vi "SIMPS 2.5.vi"() -> ()   [LabVIEW 2020]
uses:
  <vilib>/Utility/NIReport.llb/Report Type.ctl
  <vilib>/Analysis/1siggen.llb/Ramp Pattern by Samples.vi
  <vilib>/measure/maspectr.llb/FFT Spectrum (Mag-Phase) for 1 Chan.vi
  <vilib>/addons/_office/excel.llb/Excel Easy Table (num).vi
  <vilib>/Utility/NIReport.llb/NI_report.lvclass
  <vilib>/measure/NI_MABase.lvlib
  <vilib>/Analysis/NI_AALBase.lvlib
  <vilib>/Utility/NIReport.llb/NI_ReportGenerationCore.lvlib
  <vilib>/Utility/NIReport.llb/Excel/NI_Excel.lvclass
  <vilib>/addons/_office/NI_ReportGenerationToolkit.lvlib
  <vilib>/measure/NI_MAPro.lvlib
panel:
  out "Analysis Data":dynamicdata[](array[waveform])
  in  "Trigger Measurement":bool
  out "Device Mode":string
  in  "Trigger Program":bool
  in  "Generate Results Report":bool
  out "Function Generator Waveform":waveform(dbl)
  out "DUT Waveform":waveform(dbl)
  out "Gain (Multiplier)":dbl
  out "Slew Rate (V/s)":dbl
  out "Overshoot (%)":dbl
  out "Preshoot (%)":dbl
  out "Frequency (Hz) 2":dbl
  out "SINAD (dB)":dbl
  out "Amplitude (Vpk-pk)":dbl
  out "MEAN (DC V)":dbl
  out "THD (%)":dbl
  out "Negative Peak (Vpk)":dbl
  out "Positive Peak (Vpk)":dbl
  out "RMS (Vrms)":dbl
  in  "PS Update":bool
  out "Actual Voltage":dbl
  in  "PS State":bool
  out "PS Enabled":bool
  in  "Power Supply (V)":dbl=1.6 min=1.6 max=59.3
  in  "Range Selection":u8=1 min=1 max=4 step=1
  out "Current Range":u8
  in  "FG State":bool
  out "FG Enabled":bool
  in  "Duty Cycle (%)":dbl=50.0
  in  "Phase (Degrees)":dbl
  in  "DC Offset (V)":dbl min=-5.0 max=5.0 step=0.1
  in  "Frequency (Hz)":dbl=1000.0 min=1.0 max=2000000.0 step=1.0
  in  "Amplitude (V)":dbl=5.0 min=0.0 max=10.0 step=0.1
  in  "Function Selection":enum16{"Sine", "Square", "Triangle", "Ramp"}(ring)
  out "Measurement Waveforms":waveform(dbl)[](graph)
  out "FFT Magnitude":cluster{"f0":dbl, "df":dbl, "magnitude":dbl[]}(graph)
  out "FFT Phase":cluster{"f0":dbl, "df":dbl, "phase":dbl[]}(graph)
  out "Function Generator Waveform Graph":waveform(dbl)(graph)
  # "SIMPS ATE - LabVIEW Interface"
  # "Note: The device needs to be in the programming mode to program."
  # "Test Results & Analysis"
  # "Gain"
  # "Distortion Measurements"
  # "Level Measurements"
  # "Timing/Transition Measurements"
  # "DC Power Supply"
  # "The voltage entry is rounded to the nearest 10-bit value."
  # "Measurement"
  # "Select a proper range for the measurement of the DUT."
  # "1: 0-4V, 2: 4-10V, 3: 10-20V, 4: 20-60V"
  # "Function Generator"
  # "Note: The device must be programmed to change the function generator output."
  # "Eric Birtcil, Travis Draney, Nick Peck, Kyle Roy"
  # "Team Unlimited Power's Capstone Project"
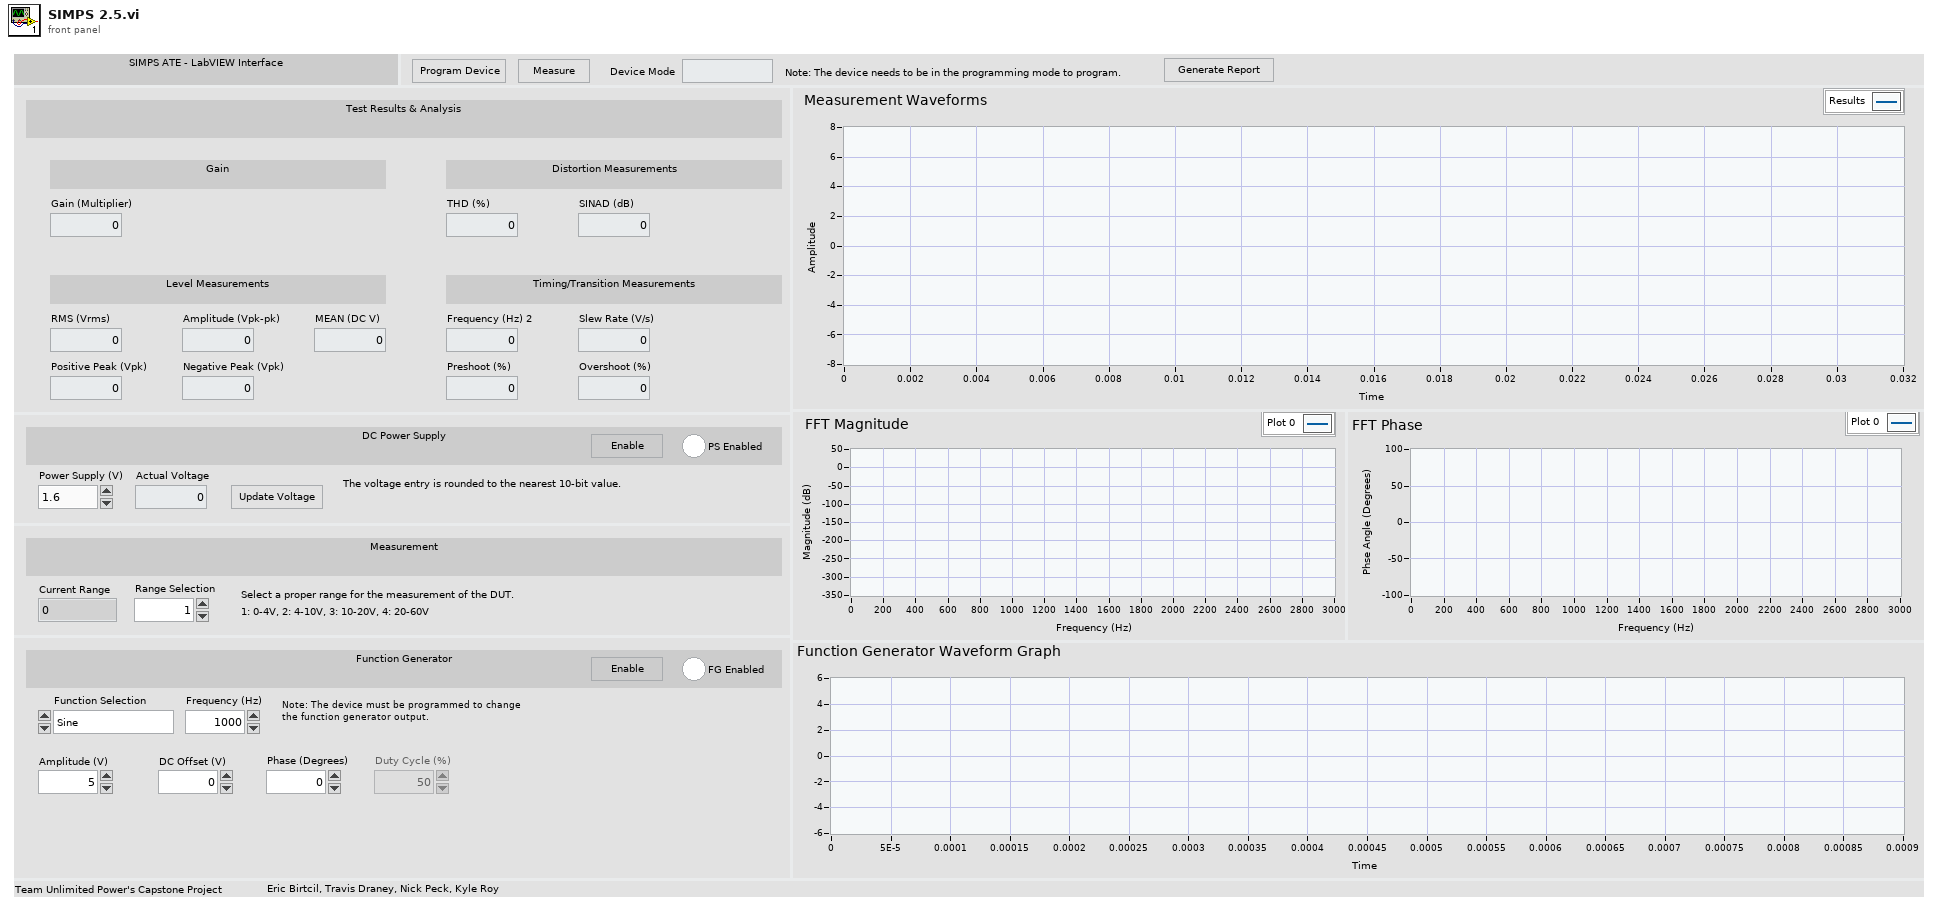
[diagram p1: front panel]
types:
  T1 = typedef "NI_ReportGenerationCore.lvlib/Report Type.ctl" = enum16{"HTML", "Word", "Excel"}
  T2 = enum8{"Enabled", "Disabled", "Disabled and Grayed Out"}
  T3 = cluster{"dB On (F)":bool, "unwrap phase (F)":bool, "convert to degree (F)":bool}
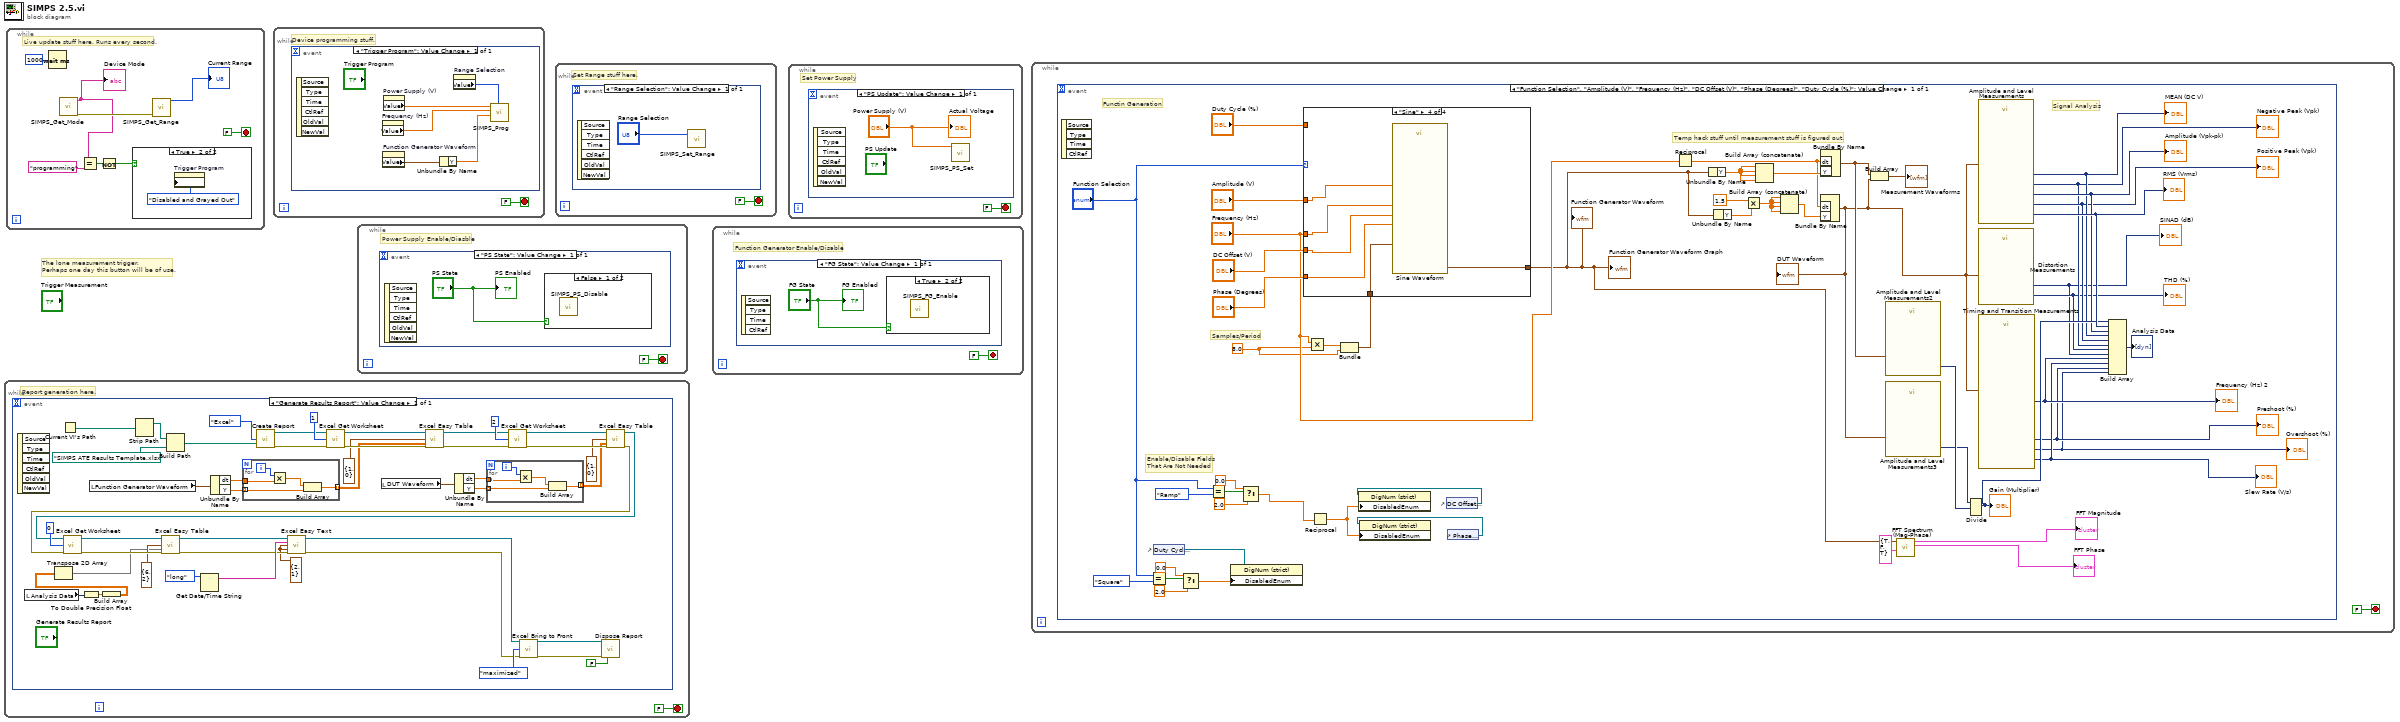
[diagram p0: block diagram]
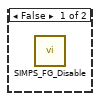
[diagram p2: hidden frame]
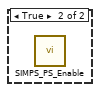
[diagram p3: hidden frame]
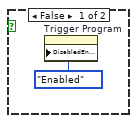
[diagram p4: hidden frame]
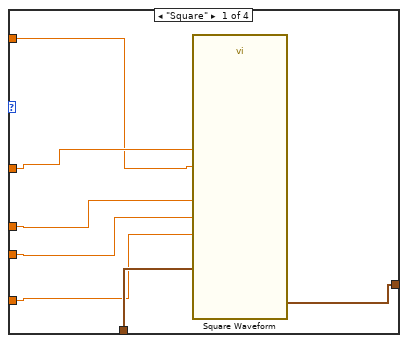
[diagram p5: hidden frame]
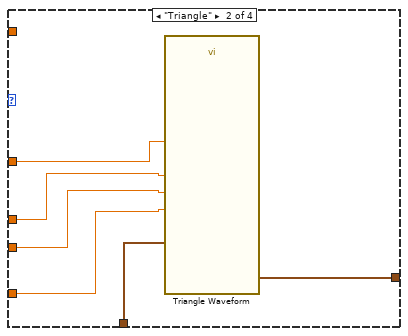
[diagram p6: hidden frame]
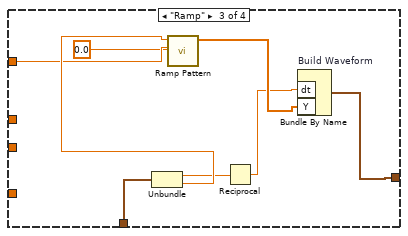
[diagram p7: hidden frame]
diagram:
  # "The lone measurement trigger.\nPerhaps one day this button will be of use."
  n1 = while {
    stop <- FALSE stop-if-true
    # "Report generation here."
    n2 = event shown="[0] \"Generate Results Report\": Value Change" {
      selector: _ -> [_]
      dyn-events: _ -> [_]
      timeout: _ -> [_]
      event "Generate Results Report": Value Change {
        w4 = cluster{"row":i32, "column":i32} {"row"=2, "column"=1} ("start (-1, -1)")
        n3 = event-data() -> ()  [unwired: 1 in, 6 out]
        n4 = local read "Analysis Data"() -> (w13:dynamicdata[])
        n5 = Current VI's Path() -> (path=w33:path)
        n6 = To Double Precision Float(number=w13) -> (double precision float=w14:dbl[])
        n7 = local read "Function Generator Waveform"() -> (w36:waveform(dbl))
        n8 = Build Array(w14) -> (w2:dbl[][])
        n9 = Transpose 2D Array(2D array=w2) -> (transposed array=w3:dbl[][])
        n10 = Strip Path(path=w33) -> (stripped path=w34:path)  [unwired: 1 out]
        n11 = Build Path(base path=w34, name or relative path=path "SIMPS ATE Results Template.xlsx") -> (appended path=w45:path)
        n12 = Get Date/Time String(date format (0)=enum16{"short", "long", "abbreviated"}."long") -> (date string=w9:string)  [unwired: 2 in, 1 out]
        n13 = Unbundle By Name(w36) -> ("dt"=w38:dbl, "Y"=w37:dbl[])
        n14 = for {
          tunnel: w38 -> [w57]
          tunnel: w37 -> [w55] mode=indexing
          tunnel: [w53] -> w30 mode=indexing
          i -> [w56]
          n15 = Multiply(x=w56, y=w57) -> (x*y=w54:dbl)
          n16 = Build Array(w54, w55) -> (w53:dbl[])
        }
        n17 = call <vilib>:"Create Report.vi"("report type"=Report_Type."Excel", "template (empty)"=w45) -> ("report out"=w43:refnum<class "NI_report.lvclass">, "error out"=w42:errorcluster)  [unwired: 12 in]
        n18 = call <vilib>:"Excel Get Worksheet.vi"("report in"=w43, "worksheet index (0)"=1, "error in (no error)"=w42) -> ("report out"=w31:refnum<class "NI_report.lvclass">, "error out"=w32:errorcluster)  [unwired: 11 in]
        n19 = local read "DUT Waveform"() -> (w19:waveform(dbl))
        n20 = call-poly <vilib>:"Excel Easy Table.vi"("report in"=w31, "start (0, 0)"=cluster{"row":i32, "column":i32} {"row"=1, "column"=0}, "text data"=w30, "error in (no error)"=w32) -> ("report out"=w21:refnum<class "NI_report.lvclass">, "error out"=w20:errorcluster)  [unwired: 7 in, 3 out]
        n21 = Unbundle By Name(w19) -> ("dt"=w28:dbl, "Y"=w27:dbl[])
        n22 = for {
          tunnel: w28 -> [w52]
          tunnel: w27 -> [w50] mode=indexing
          tunnel: [w48] -> w24 mode=indexing
          i -> [w51]
          n23 = Multiply(x=w51, y=w52) -> (x*y=w49:dbl)
          n24 = Build Array(w49, w50) -> (w48:dbl[])
        }
        n25 = call <vilib>:"Excel Get Worksheet.vi"("report in"=w21, "worksheet index (0)"=2, "error in (no error)"=w20) -> ("report out"=w25:refnum<class "NI_report.lvclass">, "error out"=w26:errorcluster)  [unwired: 11 in]
        n26 = call-poly <vilib>:"Excel Easy Table.vi"("report in"=w25, "start (0, 0)"=cluster{"row":i32, "column":i32} {"row"=1, "column"=0}, "text data"=w24, "error in (no error)"=w26) -> ("report out"=w11:refnum<class "NI_report.lvclass">, "error out"=w12:errorcluster)  [unwired: 7 in, 3 out]
        n27 = call <vilib>:"Excel Get Worksheet.vi"("report in"=w11, "worksheet index (0)"=0, "error in (no error)"=w12) -> ("report out"=w17:refnum<class "NI_report.lvclass">, "error out"=w18:errorcluster)  [unwired: 11 in]
        n28 = call-poly <vilib>:"Excel Easy Table.vi"("report in"=w17, "start (0, 0)"=cluster{"row":i32, "column":i32} {"row"=6, "column"=2}, "text data"=w3, "error in (no error)"=w18) -> ("report out"=w8:refnum<class "NI_report.lvclass">, "error out"=w7:errorcluster)  [unwired: 7 in, 3 out]
        n29 = call <vilib>:"Excel Easy Text.vi"("report in"=w8, "text"=w9, "start (-1, -1)"=w4, "end (-1, -1)"=w4, "error in (no error)"=w7) -> ("report out"=w6:refnum<class "NI_report.lvclass">, "error out"=w5:errorcluster)  [unwired: 6 in, 3 out]
        n30 = call <vilib>:"Excel Bring to Front.vi"("report in"=w6, "window state (maximized)"=enum16{"maximized", "minimized", "normal"}."maximized", "error in (no error)"=w5) -> ("report out"=w40:refnum<class "NI_report.lvclass">, "error out"=w39:errorcluster)  [unwired: 11 in]
        n31 = call-dynamic "Dispose Report.vi"("report in"=w40, "error in (no error)"=w39, "close report? (T)"=FALSE) -> ()  [unwired: 12 in, 1 out]
      }
    }
  }
  n32 = while {
    stop <- FALSE stop-if-true
    # "Live update stuff here. Runs every second."
    n33 = Wait (ms)(milliseconds to wait=u32 1000) -> ()  [unwired: 1 out]
    n34 = call "SIMPS_Get_Mode.vi"() -> ("error out"=w62:errorcluster, "String"=w61:string)  [unwired: 10 in]
    "Device Mode" <- w61
    n35 = Equal?(x=w61, y="programming") -> (x = y?=w59:bool)
    n36 = Not(x=w59) -> (.not. x?=w58:bool)
    n37 = case shown="True" w58 {
      frame False {
        n38 = property on="Trigger Program" class="Bool"("DisabledEnum"=T2."Enabled" ("Disabled")) -> ()  [unwired: 2 in, 2 out]
      }
      frame True {
        n39 = property on="Trigger Program" class="Bool"("DisabledEnum"=T2."Disabled and Grayed Out" ("Disabled")) -> ()  [unwired: 2 in, 2 out]
      }
    }
    n40 = call "SIMPS_Get_Range.vi"("error in (no error)"=w62) -> ("Numeric"=→"Current Range":u8)  [unwired: 9 in, 1 out]
  }
  n41 = while {
    stop <- FALSE stop-if-true
    # "Device programming stuff."
    n42 = event shown="[0] \"Trigger Program\": Value Change" {
      selector: _ -> [_]
      dyn-events: _ -> [_]
      timeout: _ -> [_]
      event "Trigger Program": Value Change {
        n43 = event-data() -> ()  [unwired: 1 in, 6 out]
        n44 = property on="Frequency (Hz)" class="DigNum (strict)"() -> ("Value"=w71:dbl)  [unwired: 2 in, 2 out]
        n45 = property on="Function Generator Waveform" class="WFD (strict)"() -> ("Value"=w73:waveform(dbl))  [unwired: 2 in, 2 out]
        n46 = property on="Power Supply (V)" class="DigNum (strict)"() -> ("Value"=w72:dbl)  [unwired: 2 in, 2 out]
        n47 = Unbundle By Name(w73) -> ("Y"=w69:dbl[])
        n48 = property on="Range Selection" class="DigNum (strict)"() -> ("Value"=w70:u8)  [unwired: 2 in, 2 out]
        n49 = call "SIMPS_Prog.vi"("Range"=w70, "Waveform Values"=w69, "Frequency"=w71, "PS_Voltage"=w72) -> ()  [unwired: 7 in, 1 out]
      }
    }
  }
  n50 = while {
    stop <- FALSE stop-if-true
    # "Power Supply Enable/Diasble"
    n51 = event shown="[0] \"PS State\": Value Change" {
      selector: _ -> [_]
      dyn-events: _ -> [_]
      timeout: _ -> [_]
      event "PS State": Value Change {
        n52 = event-data() -> ()  [unwired: 1 in, 6 out]
        n53 = case shown="False" "PS State" {
          frame False {
            n54 = call "SIMPS_PS_Disable.vi"() -> ()  [unwired: 11 in, 1 out]
          }
          frame True {
            n55 = call "SIMPS_PS_Enable.vi"() -> ()  [unwired: 11 in, 1 out]
          }
        }
        "PS Enabled" <- "PS State"
      }
    }
  }
  n56 = while {
    stop <- FALSE stop-if-true
    # "Set Range stuff here."
    n57 = event shown="[0] \"Range Selection\": Value Change" {
      selector: _ -> [_]
      dyn-events: _ -> [_]
      timeout: _ -> [_]
      event "Range Selection": Value Change {
        n58 = event-data() -> ()  [unwired: 1 in, 6 out]
        n59 = call "SIMPS_Set_Range.vi"("Range"="Range Selection") -> ()  [unwired: 10 in, 1 out]
      }
    }
  }
  n60 = while {
    stop <- FALSE stop-if-true
    # "Function Generator Enable/Disable"
    n61 = event shown="[0] \"FG State\": Value Change" {
      selector: _ -> [_]
      dyn-events: _ -> [_]
      timeout: _ -> [_]
      event "FG State": Value Change {
        n62 = event-data() -> ()  [unwired: 1 in, 4 out]
        n63 = case shown="True" "FG State" {
          frame False {
            n64 = call "SIMPS_FG_Disable.vi"() -> ()  [unwired: 11 in, 1 out]
          }
          frame True {
            n65 = call "SIMPS_FG_Enable.vi"() -> ()  [unwired: 11 in, 1 out]
          }
        }
        "FG Enabled" <- "FG State"
      }
    }
  }
  n66 = while {
    stop <- FALSE stop-if-true
    # "Set Power Supply"
    n67 = event shown="[0] \"PS Update\": Value Change" {
      selector: _ -> [_]
      dyn-events: _ -> [_]
      timeout: _ -> [_]
      event "PS Update": Value Change {
        n68 = event-data() -> ()  [unwired: 1 in, 6 out]
        n69 = call "SIMPS_PS_Set.vi"("PS_Voltage"="Power Supply (V)") -> ()  [unwired: 10 in, 1 out]
        "Actual Voltage" <- "Power Supply (V)"
      }
    }
  }
  n70 = while {
    stop <- FALSE stop-if-true
    n71 = event shown="[0] \"Function Selection\", \"Amplitude (V)\", \"Frequency (Hz)\", \"DC Offset (V)\", \"Phase (Degrees)\", \"Duty Cycle (%)\": Value Change" {
      selector: _ -> [_]
      dyn-events: _ -> [_]
      timeout: _ -> [_]
      event "Function Selection", "Amplitude (V)", "Frequency (Hz)", "DC Offset (V)", "Phase (Degrees)", "Duty Cycle (%)": Value Change {
        w83 = 8.0 ("Samples/Period")
        # "Temp hack stuff until measurement stuff is figured out."
        # "Samples/Period"
        # "Enable/Disable Fields\nThat Are Not Needed"
        # "Signal Analysis"
        # "Functin Generation"
        n72 = event-data() -> ()  [unwired: 1 in, 4 out]
        n73 = Equal?(x="Function Selection", y=enum16{"Sine", "Square", "Triangle", "Ramp"}."Square") -> (x = y?=w128:bool)
        n74 = control-ref of="Duty Cycle (%)"() -> (w124:refnum<vi>)
        n75 = Select(t=0.0, s=w128, f=2.0) -> (s? t:f=w123:dbl)
        n76 = Equal?(x="Function Selection", y=enum16{"Sine", "Square", "Triangle", "Ramp"}."Ramp") -> (x = y?=w121:bool)
        n77 = property class="DigNum (strict)"(reference=w124, "DisabledEnum"=w123) -> ()  [unwired: 1 in, 2 out]
        n78 = Select(t=0.0, s=w121, f=2.0) -> (s? t:f=w117:dbl)
        n79 = Multiply(x="Frequency (Hz)", y=w83) -> (x*y=w133:dbl)
        n80 = Reciprocal(x=w117) -> (1/x=w116:dbl)
        n81 = Bundle(w133, "Samples/Period"=w83) -> (w134:cluster{dbl, "Samples/Period":dbl})  [unwired: 1 in]
        n82 = case shown="\"Sine\"" "Function Selection" {
          tunnel: [w141 w147 w155 w156] -> w85
          tunnel: "Amplitude (V)" -> [w136 w146 w149 w157]
          tunnel: "Frequency (Hz)" -> [w137 w145 _ w158]
          tunnel: "DC Offset (V)" -> [w138 w144 _ w159]
          tunnel: "Phase (Degrees)" -> [w139 w143 _ w160]
          tunnel: w134 -> [w140 w142 w154 w161]
          tunnel: "Duty Cycle (%)" -> [w135 _ _ _]
          frame "Square" {
            n83 = call <vilib>:"Square Waveform.vi"("duty cycle (%)"=w135, "offset"=w138, "sampling info"=w140, "phase"=w139, "amplitude"=w136, "frequency"=w137) -> ("signal out"=w141:waveform(dbl))  [unwired: 4 in, 1 out]
          }
          frame "Triangle" {
            n84 = call <vilib>:"Triangle Waveform.vi"("offset"=w144, "sampling info"=w142, "phase"=w143, "amplitude"=w146, "frequency"=w145) -> ("signal out"=w147:waveform(dbl))  [unwired: 5 in, 1 out]
          }
          frame "Ramp" {
            n85 = Unbundle(w154) -> (w151:dbl, "Samples/Period"=w153:dbl)
            n86 = call-poly <vilib>:"Ramp Pattern.vi"("start"=0.0, "end"=w149, "samples"=w153) -> ("Ramp Pattern"=w152:dbl[])  [unwired: 7 in, 1 out]
            n87 = Reciprocal(x=w151) -> (1/x=w150:dbl)
            n88 = Bundle By Name "Build Waveform"("dt"=w150, "Y"=w152) -> (w155:waveform(dbl))  [unwired: 1 in]
          }
          frame "Sine" {
            n89 = call <vilib>:"Sine Waveform.vi"("offset"=w159, "sampling info"=w161, "phase"=w160, "amplitude"=w157, "frequency"=w158) -> ("signal out"=w156:waveform(dbl))  [unwired: 5 in, 1 out]
          }
        }
        "Function Generator Waveform Graph" <- w85
        "Function Generator Waveform" <- w85
        n90 = control-ref of="DC Offset (V)"() -> (w115:refnum<vi>)
        n91 = property class="DigNum (strict)"(reference=w115, "DisabledEnum"=w116) -> ()  [unwired: 1 in, 2 out]
        n92 = control-ref of="Phase (Degrees)"() -> (w114:refnum<vi>)
        n93 = property class="DigNum (strict)"(reference=w114, "DisabledEnum"=w116) -> ()  [unwired: 1 in, 2 out]
        n94 = Reciprocal(x="Frequency (Hz)") -> (1/x=w106:dbl)
        n95 = Unbundle By Name(w85) -> ("Y"=w111:dbl[])
        n96 = Unbundle By Name(w85) -> ("Y"=w110:dbl[])
        n97 = Multiply(x=1.5, y=w110) -> (x*y=w108:dbl[])
        n98 = Build Array (concatenate)(w111, w111, w111, w111) -> (w112:dbl[])
        n99 = Build Array (concatenate)(w108, w108, w108, w108) -> (w105:dbl[])
        n100 = Bundle By Name("dt"=w106, "Y"=w105) -> (w88:waveform(dbl))  [unwired: 1 in]
        "DUT Waveform" <- w88
        n101 = Bundle By Name("dt"=w106, "Y"=w112) -> (w104:waveform(dbl))  [unwired: 1 in]
        n102 = Build Array(w104, w88) -> (→"Measurement Waveforms":waveform(dbl)[])
        n103 = call "Amplitude and Level Measurements2"("Signals"=w104) -> ("Peak to Peak"=w103:dynamicdata)  [unwired: 13 in, 1 out]
        n104 = call "Amplitude and Level Measurements3"("Signals"=w88) -> ("Peak to Peak"=w102:dynamicdata)  [unwired: 13 in, 1 out]
        n105 = call-poly <vilib>:"FFT Spectrum (Mag-Phase).vi"("view"=T3 {"dB On (F)"=TRUE, "unwrap phase (F)"=FALSE, "convert to degree (F)"=TRUE}, "time signal"=w85) -> ("phase"=→"FFT Phase":cluster{"f0":dbl, "df":dbl, "phase":dbl[]}, "magnitude"=→"FFT Magnitude":cluster{"f0":dbl, "df":dbl, "magnitude":dbl[]})  [unwired: 5 in, 3 out]
        n106 = Divide(1:w103, 2:w102) -> (0:w100:dynamicdata)  [unwired: 1 in, 1 out]
        "Gain (Multiplier)" <- w100
        n107 = call "Amplitude and Level Measurements"("Signals"=w88) -> ("Mean (DC)"=w98:dynamicdata, "RMS"=w101:dynamicdata, "Negative Peak"=w96:dynamicdata, "Positive Peak"=w97:dynamicdata, "Peak to Peak"=w99:dynamicdata)  [unwired: 9 in, 1 out]
        "RMS (Vrms)" <- w101
        "Positive Peak (Vpk)" <- w97
        "Negative Peak (Vpk)" <- w96
        "MEAN (DC V)" <- w98
        "Amplitude (Vpk-pk)" <- w99
        n108 = call "Distortion Measurements"("Signals"=w88) -> ("SINAD (dB)"=w94:dynamicdata, "THD"=w95:dynamicdata)  [unwired: 8 in, 1 out]
        "THD (%)" <- w95
        "SINAD (dB)" <- w94
        n109 = call "Timing and Transition Measurements"("Signals"=w88) -> ("Frequency"=w93:dynamicdata, "Preshoot"=w91:dynamicdata, "Overshoot"=w90:dynamicdata, "Slew Rate"=w92:dynamicdata)  [unwired: 3 in, 4 out]
        "Overshoot (%)" <- w90
        "Slew Rate (V/s)" <- w92
        "Preshoot (%)" <- w91
        "Frequency (Hz) 2" <- w93
        n110 = Build Array(w100, w101, w99, w98, w97, w96, w95, w94, w93, w92, w91, w90) -> (→"Analysis Data":dynamicdata[])
      }
    }
  }
